vi "Test2_3a.vi"(7 "Report Enable":bool=TRUE, 8 "error in":errorcluster, 9 "Cycles Burst":i32=10000, 11 "Instrument VISA in":T1={"AWG VISA"="81160A", "Oscilloscope  VISA "="labosc4", "Integration Board IP"="172.16.7.43", "connection ID"=refnum, "report out"=refnum, "report file path"=path "D:/CTA/Data_test/test3a"}) -> (0 "error out":errorcluster, 3 "Instrument VISA out":T1={"AWG VISA"="81160A", "Oscilloscope  VISA "="DSO80204B", "Integration Board IP"="172.16.7.43", "connection ID"=refnum, "report out"=refnum, "report file path"=path "D:/CTA/LevelTriggerBoardTest/TestsData/sumtrigger_delay/dataruben"})   [LabVIEW 2009]
uses:
  <vilib>/Utility/NIReport.llb/NI_report.lvclass
  <vilib>/Utility/NIReport.llb/HTML/NI_HTML.lvclass
  <instrlib>/Agilent 8000 Series/Public/Configure/Configure Math (Binary Operation).vi
  <instrlib>/Agilent 81150/Agilent 81150.lvlib
  <instrlib>/Agilent 8000 Series/Agilent 8000 Series.lvlib
panel:
  in  "Voltages comprobation 2":dbl[](array[numeric])=[0.05, 0.1, 0.2, 0.3, 0.35, 0.4, 0.45, 0.5, 0.55, 0.6, 0.7, 0.8, 0.9, 1.0, 1.2, 1.5, 1.8, 2.0]
  in  "Voltages comprobation":dbl[](array[numeric])=[0.05, 0.1, 0.2, 0.3, 0.35, 0.4, 0.45, 0.5, 0.55, 0.6, 0.7, 0.8, 0.9, 1.0, 1.2, 1.5, 1.8, 2.0]
  in  "cliipping":i32[](array[numeric])=[504, 502, 520, 505, 498, 488, 458]
  in  "attenuation":i32[](array[numeric])=[1473, 1472, 1442, 1475, 1463, 1454, 1478]
  in  "Channels":i32[](array[numeric])=[0, 1, 2, 3, 4, 5, 6]
  in  "Quantity of measurements":u32=10
  in  "Save NOW!":bool
  in  "End 2":bool=TRUE
  out "Data output":dbl[][](array[numeric])=[[1.0, 1.0, 2200.0, 200.0, 0.0, 0.26, nan, 1.00955e-08, nan, 2.8861e-09, nan, 0.961, nan], [1.0, 1.0, 2200.0, 200.0, 1.0, 0.261, nan, 1.0146e-08, nan, 2.9059e-09, nan, 0.961, nan]]
  out "Measurement":dbl=0.261
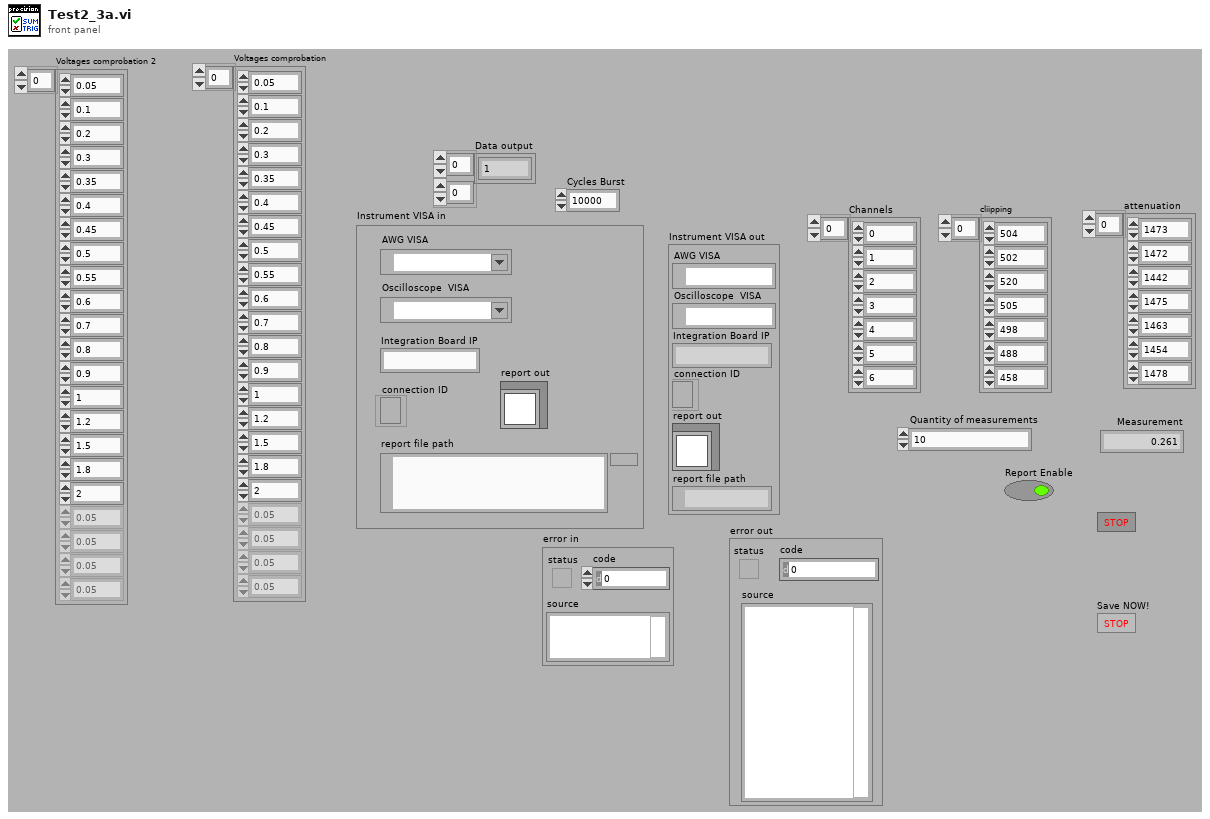
[diagram p1: front panel]
types:
  T1 = cluster{"AWG VISA":refnum<visa-resource-name>, "Oscilloscope  VISA ":refnum<visa-resource-name>, "Integration Board IP":string, "connection ID":refnum<k5>, "report out":refnum<class "NI_report.lvclass">, "report file path":path}
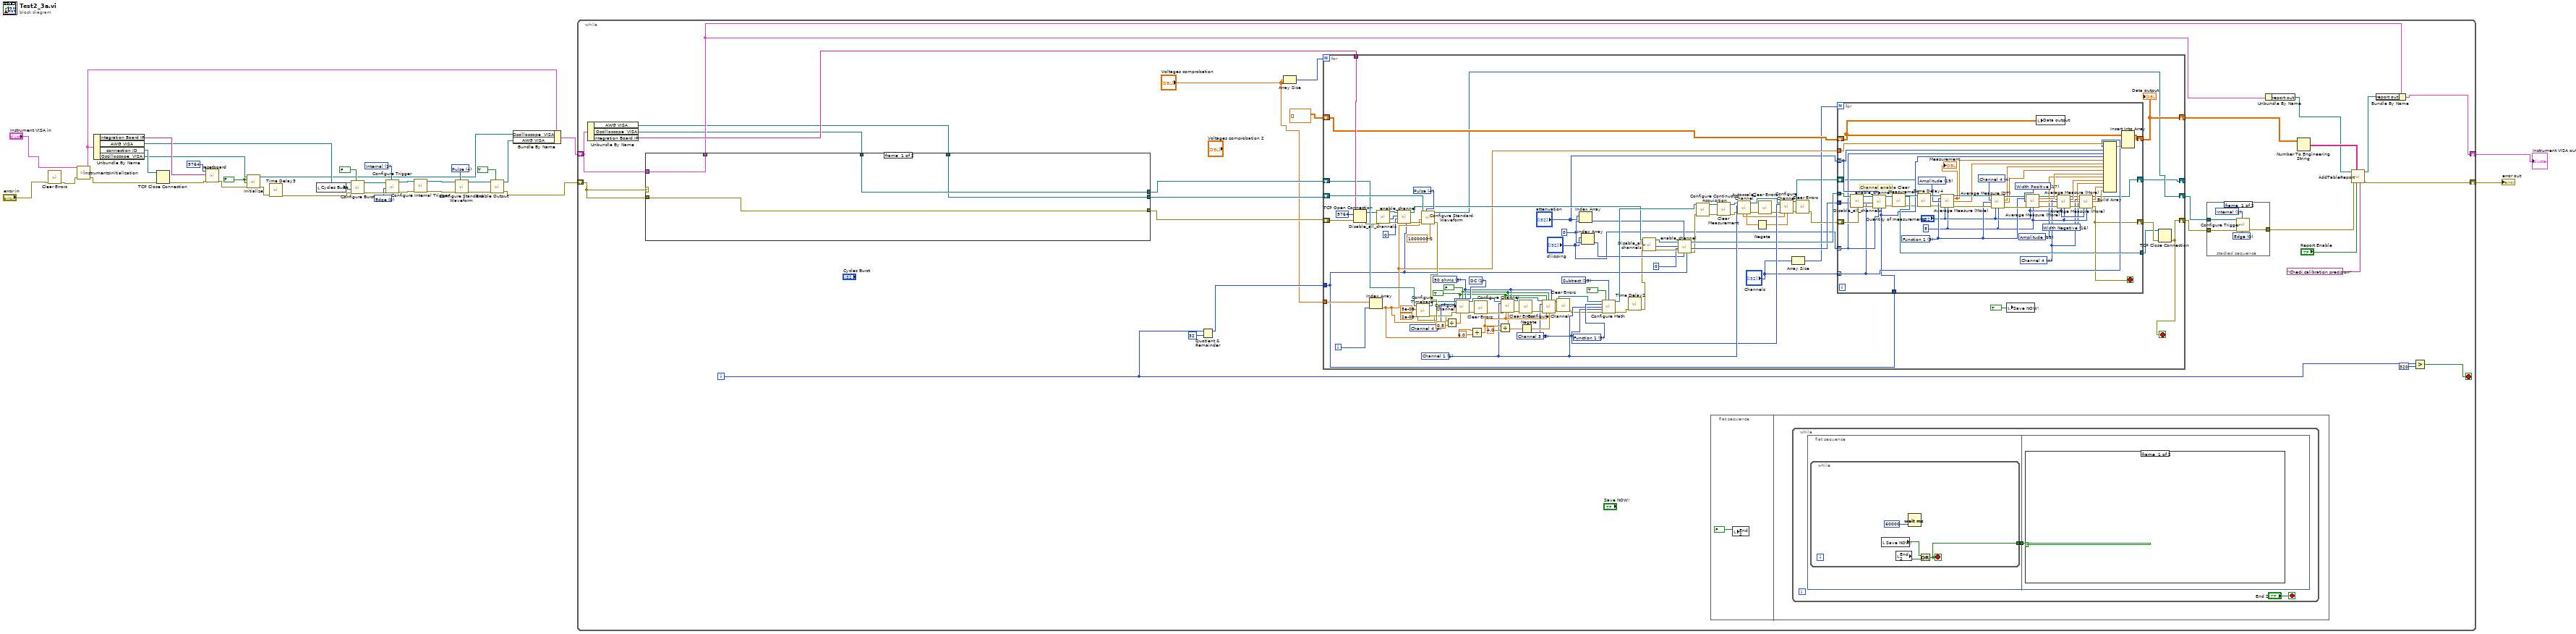
[diagram p0: block diagram]
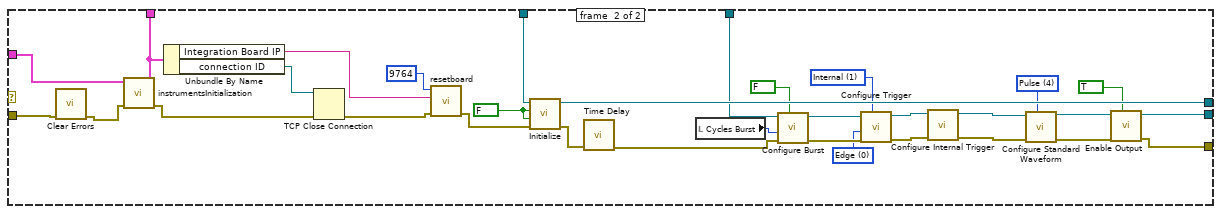
[diagram p2: hidden frame]
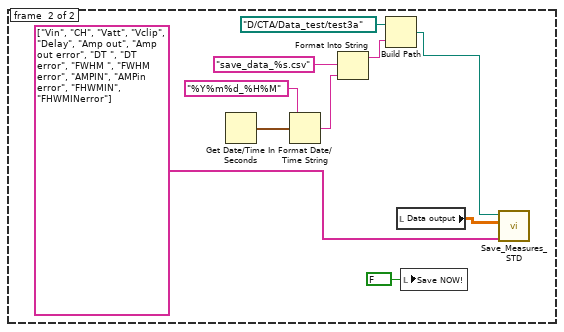
[diagram p3: hidden frame]
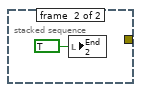
[diagram p4: hidden frame]
diagram:
  w18 = u16 1 items=["Immediate", "Internal", "External", "Software Trigger Function"] ("Trigger Source (0: Immediate)")
  w19 = u16 0 items=["Edge", "Level"] ("Trigger Mode (0: Edge)")
  w26 = u16 4 items=["Sine", "Square", "Ramp Up", "Ramp Down", "Pulse", "Noise", "DC"] ("Waveform (0: Sine)")
  w31 = FALSE ("ID Query (True)")
  n1 = call <vilib>:"Clear Errors.vi"("error in (no error)"="error in") -> ("error out"=w28:errorcluster)  [unwired: 6 in]
  n2 = call "instrumentsInitialization.vi"("error in"=w28, "Instrument VISA in"="Instrument VISA in") -> ("error out"=w11:errorcluster, "Instrument VISA out"=w4:T1)  [unwired: 8 in]
  n3 = Unbundle By Name(w4) -> ("Integration Board IP"=w33:string, "AWG VISA"=w6:refnum<visa-resource-name>, "connection ID"=w12:refnum<k5>, "Oscilloscope  VISA"=w7:refnum<visa-resource-name>)
  n4 = TCP Close Connection(connection ID=w12, error in (no error)=w11) -> (error out=w10:errorcluster)  [unwired: 1 in, 1 out]
  n5 = call "resetboard.vi"("error in (no error)"=w10, "address"=w33, "remote port or service name"=u16 9764) -> ("error out"=w30:errorcluster)  [unwired: 7 in, 1 out]
  n6 = call <instrlib>:"Initialize.vi"("error in (no error)"=w30, "Reset (True)"=w31, "ID Query (True)"=w31, "VISA resource name"=w7) -> ("error out"=w29:errorcluster, "VISA resource name out"=w3:refnum<visa-resource-name>)  [unwired: 6 in]
  n7 = call "Time Delay3"("error in (no error)"=w29) -> ("error out"=w13:errorcluster)  [unwired: 10 in]
  n8 = local read "Cycles Burst"() -> (w22:i32)
  n9 = call <instrlib>:"Configure Burst.vi"("Enable Burst (F: Disable)"=FALSE, "error in (no error)"=w13, "Burst Count (2)"=w22, "VISA resource name"=w6) -> ("error out"=w21:errorcluster, "VISA resource name out"=w20:refnum<visa-resource-name>)  [unwired: 6 in]
  n10 = call <instrlib>:"Configure Trigger.vi"("Trigger Source (0: Immediate)"=w18, "error in (no error)"=w21, "Trigger Mode (0: Edge)"=w19, "VISA resource name"=w20) -> ("error out"=w17:errorcluster, "VISA resource name out"=w16:refnum<visa-resource-name>)  [unwired: 6 in]
  n11 = call <instrlib>:"Configure Internal Trigger.vi"("error in (no error)"=w17, "VISA resource name"=w16) -> ("error out"=w14:errorcluster, "VISA resource name out"=w15:refnum<visa-resource-name>)  [unwired: 8 in]
  n12 = call <instrlib>:"Configure Standard Waveform.vi"("Waveform (0: Sine)"=w26, "error in (no error)"=w14, "VISA resource name"=w15) -> ("error out"=w25:errorcluster, "VISA resource name out"=w24:refnum<visa-resource-name>)  [unwired: 7 in]
  n13 = call <instrlib>:"Enable Output.vi"("Enable Output (T: Enable)"=TRUE, "error in (no error)"=w25, "VISA resource name"=w24) -> ("error out"=w5:errorcluster, "VISA resource name out"=w2:refnum<visa-resource-name>)  [unwired: 7 in]
  n14 = Bundle By Name(cluster=w4, "Oscilloscope  VISA"=w3, "AWG VISA"=w2) -> (w1:T1)
  n15 = while {
    shift-right: [w48] -> w35
    shift-left: w5 -> [w40]
    shift-right: [w44] -> w34
    shift-left: w1 -> [w46]
    i -> [w51]
    stop <- w53 stop-if-true
    n16 = Unbundle By Name(w46) -> ("AWG VISA"=w39:refnum<visa-resource-name>, "Oscilloscope  VISA"=w42:refnum<visa-resource-name>, "Integration Board IP"=w47:string)
    n17 = case shown="Error" w40 {
      tunnel: w46 -> [w67 w99]
      tunnel: w40 -> [w66 w90]
      tunnel: [w67 w98] -> w45
      tunnel: [w66 w72] -> w37
      tunnel: w42 -> [w65 w95]
      tunnel: [w65 w94] -> w41
      tunnel: w39 -> [w64 w74]
      tunnel: [w64 w73] -> w38
      frame #0 {
      }
      frame #1 {
        w79 = u16 1 items=["Immediate", "Internal", "External", "Software Trigger Function"] ("Trigger Source (0: Immediate)")
        w80 = u16 0 items=["Edge", "Level"] ("Trigger Mode (0: Edge)")
        w87 = u16 4 items=["Sine", "Square", "Ramp Up", "Ramp Down", "Pulse", "Noise", "DC"] ("Waveform (0: Sine)")
        w93 = FALSE ("ID Query (True)")
        n18 = call <vilib>:"Clear Errors.vi"("error in (no error)"=w90) -> ("error out"=w89:errorcluster)  [unwired: 6 in]
        n19 = call "instrumentsInitialization.vi"("error in"=w89, "Instrument VISA in"=w99) -> ("error out"=w69:errorcluster, "Instrument VISA out"=w98:T1)  [unwired: 8 in]
        n20 = Unbundle By Name(w98) -> ("Integration Board IP"=w97:string, "connection ID"=w70:refnum<k5>)
        n21 = TCP Close Connection(connection ID=w70, error in (no error)=w69) -> (error out=w68:errorcluster)  [unwired: 1 in, 1 out]
        n22 = call "resetboard.vi"("error in (no error)"=w68, "address"=w97, "remote port or service name"=u16 9764) -> ("error out"=w92:errorcluster)  [unwired: 7 in, 1 out]
        n23 = call <instrlib>:"Initialize.vi"("error in (no error)"=w92, "Reset (True)"=w93, "ID Query (True)"=w93, "VISA resource name"=w95) -> ("error out"=w91:errorcluster, "VISA resource name out"=w94:refnum<visa-resource-name>)  [unwired: 6 in]
        n24 = call "Time Delay"("error in (no error)"=w91) -> ("error out"=w71:errorcluster)  [unwired: 10 in]
        n25 = local read "Cycles Burst"() -> (w83:i32)
        n26 = call <instrlib>:"Configure Burst.vi"("Enable Burst (F: Disable)"=FALSE, "error in (no error)"=w71, "Burst Count (2)"=w83, "VISA resource name"=w74) -> ("error out"=w82:errorcluster, "VISA resource name out"=w81:refnum<visa-resource-name>)  [unwired: 6 in]
        n27 = call <instrlib>:"Configure Trigger.vi"("Trigger Source (0: Immediate)"=w79, "error in (no error)"=w82, "Trigger Mode (0: Edge)"=w80, "VISA resource name"=w81) -> ("error out"=w78:errorcluster, "VISA resource name out"=w77:refnum<visa-resource-name>)  [unwired: 6 in]
        n28 = call <instrlib>:"Configure Internal Trigger.vi"("error in (no error)"=w78, "VISA resource name"=w77) -> ("error out"=w75:errorcluster, "VISA resource name out"=w76:refnum<visa-resource-name>)  [unwired: 8 in]
        n29 = call <instrlib>:"Configure Standard Waveform.vi"("Waveform (0: Sine)"=w87, "error in (no error)"=w75, "VISA resource name"=w76) -> ("error out"=w86:errorcluster, "VISA resource name out"=w85:refnum<visa-resource-name>)  [unwired: 7 in]
        n30 = call <instrlib>:"Enable Output.vi"("Enable Output (T: Enable)"=TRUE, "error in (no error)"=w86, "VISA resource name"=w85) -> ("error out"=w72:errorcluster, "VISA resource name out"=w73:refnum<visa-resource-name>)  [unwired: 7 in]
      }
    }
    n31 = Quotient & Remainder(x=w51, y=32) -> (x-y*floor(x/y)=w49:i32)  [unwired: 1 out]
    n32 = Array Size(array="Voltages comprobation") -> (size(s)=w54:i32)
    n33 = for {
      N: w54 -> [_]
      shift-right: [w204] -> w63
      shift-left: w37 -> [w207]
      tunnel: w47 -> [w206]
      shift-right: [w164] -> w58
      shift-left: dbl[][] [] -> [w167]
      tunnel: "Voltages comprobation" -> [w163]
      tunnel: w49 -> [w132]
      shift-right: [w131] -> w43
      shift-left: w38 -> [w210]
      shift-right: [w130] -> _
      shift-left: w41 -> [w201]
      i -> [w209]
      stop <- w204 stop-if-true
      w139 = 0 ("index")
      w181 = TRUE ("Enable Channel (Enable)")
      w183 = FALSE ("BW Limit 20MHz (Disable)")
      w182 = u32 0 items=["50 ohms", "1 Mohms"] ("Input Impedance (1: 1 Mohms)")
      w191 = 4 items=["Channel 1"=1, "Channel 2"=2, "Channel 3"=3, "Channel 4"=4] ("Channel (1: Channel 1)")
      w192 = 1 items=["AC", "DC"] ("Vertical Coupling (1: DC)")
      w196 = u16 5 items=["Function 1"=5, "Function 2"=6, "Function 3"=7, "Function 4"=8] ("Math Channel (5: Function 1)")
      w197 = u16 15 items=["Add"=12, "Divide"=13, "Multiply"=14, "Subtract"=15, "Common Mode"=16, "Versus"=17] ("Math Operation (12: Add)")
      w166 = 1 items=["Channel 1"=1, "Channel 2"=2, "Channel 3"=3, "Channel 4"=4] ("Channel (1: Channel 1)")
      w165 = 3 items=["Channel 1"=1, "Channel 2"=2, "Channel 3"=3, "Channel 4"=4] ("Channel (1: Channel 1)")
      w211 = u16 4 items=["Sine", "Square", "Ramp Up", "Ramp Down", "Pulse", "Noise", "DC"] ("Waveform (0: Sine)")
      n34 = TCP Open Connection(address=w206, remote port or service name=u16 9764, error in (no error)=w207) -> (connection ID=w178:refnum<k5>, error out=w179:errorcluster)  [unwired: 2 in]
      n35 = Index Array(array=w163, index=w209) -> (element=w162:dbl)
      n36 = call "Disable_all_channels.vi"("error in"=w179, "connection ID"=w178) -> ("error out"=w174:errorcluster, "id_out"=w173:i32, "connection ID out"=w176:refnum<k5>)  [unwired: 7 in]
      n37 = call "enable_channel.vi"("Delay"=w132, "error in"=w174, "Channel"=u16 0 ("remote port or service name"), "id_in"=w173, "connection ID"=w176) -> ("error out"=w175:errorcluster, "connection ID out"=w177:refnum<k5>)  [unwired: 4 in, 1 out]
      n38 = call <instrlib>:"Configure Standard Waveform.vi"("Frequency (1000.0 Hz)"=1000000.0, "Waveform (0: Sine)"=w211, "error in (no error)"=w175, "Amplitude (1.0 Vpp)"=w162, "VISA resource name"=w210) -> ("error out"=w200:errorcluster, "VISA resource name out"=w131:refnum<visa-resource-name>)  [unwired: 5 in]
      n39 = call <instrlib>:"Configure Timebase.vi"("error in (no error)"=w200, "Position (0.0 s)"=2e-08, "Timebase (0.005 s)"=5e-08, "VISA resource name"=w201) -> ("error out"=w193:errorcluster, "VISA resource name out"=w194:refnum<visa-resource-name>)  [unwired: 6 in]
      n40 = Divide(x=w162, y=0.5) -> (x/y=w160:dbl)
      n41 = call <instrlib>:"Configure Channel.vi"("VISA resource name"=w194, "Enable Channel (Enable)"=w181, "BW Limit 20MHz (Disable)"=w183, "Input Impedance (1: 1 Mohms)"=w182, "Channel (1: Channel 1)"=w191, "Vertical Coupling (1: DC)"=w192, "error in (no error)"=w193, "Vertical Range (2.0 V)"=w160) -> ("VISA resource name out"=w189:refnum<visa-resource-name>, "error out"=w190:errorcluster)  [unwired: 6 in]
      n42 = Divide(x=w162, y=6.0) -> (x/y=w171:dbl)
      n43 = call <vilib>:"Clear Errors.vi"("error in (no error)"=w190) -> ("error out"=w186:errorcluster)  [unwired: 6 in]
      n44 = Divide(x=w171, y=4.0) -> (x/y=w168:dbl)
      n45 = call <instrlib>:"Configure Channel.vi"("VISA resource name"=w189, "Enable Channel (Enable)"=w181, "BW Limit 20MHz (Disable)"=w183, "Input Impedance (1: 1 Mohms)"=w182, "Channel (1: Channel 1)"=w166, "error in (no error)"=w186, "Vertical Range (2.0 V)"=w171, "Vertical Offset (0.0 V)"=w168) -> ("VISA resource name out"=w188:refnum<visa-resource-name>, "error out"=w185:errorcluster)  [unwired: 6 in]
      n46 = call <vilib>:"Clear Errors.vi"("error in (no error)"=w185) -> ("error out"=w184:errorcluster)  [unwired: 6 in]
      n47 = Negate(x=w168) -> (-x=w169:dbl)
      n48 = call <instrlib>:"Configure Channel.vi"("VISA resource name"=w188, "Enable Channel (Enable)"=w181, "BW Limit 20MHz (Disable)"=w183, "Input Impedance (1: 1 Mohms)"=w182, "Channel (1: Channel 1)"=w165, "error in (no error)"=w184, "Vertical Range (2.0 V)"=w171, "Vertical Offset (0.0 V)"=w169) -> ("VISA resource name out"=w187:refnum<visa-resource-name>, "error out"=w126:errorcluster)  [unwired: 6 in]
      n49 = call <vilib>:"Clear Errors.vi"("error in (no error)"=w126) -> ("error out"=w125:errorcluster)  [unwired: 6 in]
      n50 = Index Array(array="attenuation", index=w139) -> (element=w137:i32)
      n51 = Index Array(array="cliipping", index=w139) -> (element=w138:i32)
      n52 = call-poly <instrlib>:"Configure Math.vi"("VISA resource name"=w187, "Enable Math Channel (T:Enable)"=TRUE, "Math Operation (12: Add)"=w197, "Math Channel (5: Function 1)"=w196, "Math Operand (1: Channel 1)"=w166, "Math Operand (2: Channel 2)"=w165, "error in (no error)"=w125) -> ("VISA resource name out"=w199:refnum<visa-resource-name>, "error out"=w127:errorcluster)  [unwired: 7 in]
      n53 = call "Time Delay2"("error in (no error)"=w127) -> ("error out"=w128:errorcluster)  [unwired: 10 in]
      n54 = call "Disable_all_channels.vi"("error in"=w128, "connection ID"=w177) -> ("error out"=w159:errorcluster, "id_out"=w156:i32, "connection ID out"=w158:refnum<k5>)  [unwired: 7 in]
      n55 = call "enable_channel.vi"("Delay"=w132, "V clip"=w138, "V att"=w137, "error in"=w159, "Channel"=u32 0 ("Max Errors"), "id_in"=w156, "connection ID"=w158) -> ("error out"=w143:errorcluster, "id_out"=w154:i32, "connection ID out"=w157:refnum<k5>)  [unwired: 2 in]
      n56 = call <instrlib>:"Configure Continuous Acquisition.vi"("error in (no error)"=w143, "VISA resource name"=w199) -> ("error out"=w142:errorcluster, "VISA resource name out"=w144:refnum<visa-resource-name>)  [unwired: 8 in]
      n57 = call <instrlib>:"Clear Measurement.vi"("error in (no error)"=w142, "VISA resource name"=w144) -> ("error out"=w146:errorcluster, "VISA resource name out"=w145:refnum<visa-resource-name>)  [unwired: 8 in]
      n58 = call "Autoscale_Channel.vi"("error in"=w146, "Channel"=w166, "VISA resource name"=w145) -> ("error out"=w148:errorcluster, "VISA resource name out"=w153:refnum<visa-resource-name>, "Offset"=w133:dbl, "VerticalRange"=w152:dbl)  [unwired: 5 in]
      n59 = Negate(x=w133) -> (-x=w134:dbl)
      n60 = call <vilib>:"Clear Errors.vi"("error in (no error)"=w148) -> ("error out"=w149:errorcluster)  [unwired: 6 in]
      n61 = call <instrlib>:"Configure Channel.vi"("VISA resource name"=w153, "Channel (1: Channel 1)"=w165, "error in (no error)"=w149, "Vertical Range (2.0 V)"=w152, "Vertical Offset (0.0 V)"=w134) -> ("VISA resource name out"=w129:refnum<visa-resource-name>, "error out"=w150:errorcluster)  [unwired: 9 in]
      n62 = Array Size(array="Channels") -> (size(s)=w140:i32)
      n63 = call <vilib>:"Clear Errors.vi"("error in (no error)"=w150) -> ("error out"=w151:errorcluster)  [unwired: 6 in]
      n64 = for {
        N: w140 -> [_]
        shift-right: [w225] -> w205
        shift-left: w151 -> [w258]
        tunnel: w157 -> [w259]
        tunnel: [w261] -> w203
        tunnel: w162 -> [w255]
        shift-right: [w253] -> w164
        shift-left: w167 -> [w235]
        tunnel: "attenuation" -> [w238] mode=indexing
        tunnel: "cliipping" -> [w237] mode=indexing
        tunnel: w154 -> [w236]
        tunnel: "Channels" -> [w229] mode=indexing
        tunnel: w132 -> [w227]
        shift-right: [w217] -> w130
        shift-left: w129 -> [w216]
        stop <- w225 stop-if-true
        w218 = 16 items=["Rise Time", "Fall Time", "Frequency", "Period", "Voltage RMS(AC)", "Voltage RMS(DC)", "Voltage RMS (AC,cycle)", "Voltage RMS (DC,cycle)", "Voltage Max", "Voltage Min", "Voltage Middle", "Voltage Vpp", "Voltage High", "Voltage Low", "Voltage Average", "Voltage Average (cycle)", "Width Negative", "Width Positive", "Duty Cycle Positive", "Amplitude", "Overshoot", "Preshoot", "Voltage Base", "Voltage Upper", "Time Max", "Time Min", "Color Grade Crossing", "Color Grade Eye Width", "Color Grade Eye Height", "Color Grade Eye Q-Factory", "Color Grade Eye Duty Cycle Distortion(Percent)", "Color Grade Eye Duty Cycle Distortion(Time)", "Color Grade Eye Jitter(PP)", "Color Grade Eye Width(RMS)", "Cycle-cycle Duty Jitter(Rising)", "Cycle-cycle Duty Jitter(Falling)", "Cycle-cycle Jitter(Rising)", "Cycle-cycle Jitter(Falling)", "Cycle-cycle - Width", "Cycle-cycle + Width", "Date Rate", "Unit Interval", "FFT Delta Frequency", "FFT Delta Magnitude", "FFT Frequency", "FFT Magnitude", "Slew Rate", "Area (Entire Display)", "Area(Single Cycle)", "Duty Cycle (Rising)", "Duty Cycle (Falling)"] ("Measurement Function (0: Rise Time)")
        w219 = 4 items=["Channel 1"=1, "Channel 2"=2, "Channel 3"=3, "Channel 4"=4, "Function 1"=5, "Function 2"=6, "Function 3"=7, "Function 4"=8, "Memory 1"=9, "Memory 2"=10, "Memory 3"=11, "Memory 4"=12] ("Channel (1: Channel 1)")
        w233 = 19 items=["Rise Time", "Fall Time", "Frequency", "Period", "Voltage RMS(AC)", "Voltage RMS(DC)", "Voltage RMS (AC,cycle)", "Voltage RMS (DC,cycle)", "Voltage Max", "Voltage Min", "Voltage Middle", "Voltage Vpp", "Voltage High", "Voltage Low", "Voltage Average", "Voltage Average (cycle)", "Width Negative", "Width Positive", "Duty Cycle Positive", "Amplitude", "Overshoot", "Preshoot", "Voltage Base", "Voltage Upper", "Time Max", "Time Min", "Color Grade Crossing", "Color Grade Eye Width", "Color Grade Eye Height", "Color Grade Eye Q-Factory", "Color Grade Eye Duty Cycle Distortion(Percent)", "Color Grade Eye Duty Cycle Distortion(Time)", "Color Grade Eye Jitter(PP)", "Color Grade Eye Width(RMS)", "Cycle-cycle Duty Jitter(Rising)", "Cycle-cycle Duty Jitter(Falling)", "Cycle-cycle Jitter(Rising)", "Cycle-cycle Jitter(Falling)", "Cycle-cycle - Width", "Cycle-cycle + Width", "Date Rate", "Unit Interval", "FFT Delta Frequency", "FFT Delta Magnitude", "FFT Frequency", "FFT Magnitude", "Slew Rate", "Area (Entire Display)", "Area(Single Cycle)", "Duty Cycle (Rising)", "Duty Cycle (Falling)"] ("Measurement Function (0: Rise Time)")
        w221 = u32 5 ("Max Errors")
        w249 = 17 items=["Rise Time", "Fall Time", "Frequency", "Period", "Voltage RMS(AC)", "Voltage RMS(DC)", "Voltage RMS (AC,cycle)", "Voltage RMS (DC,cycle)", "Voltage Max", "Voltage Min", "Voltage Middle", "Voltage Vpp", "Voltage High", "Voltage Low", "Voltage Average", "Voltage Average (cycle)", "Width Negative", "Width Positive", "Duty Cycle Positive", "Amplitude", "Overshoot", "Preshoot", "Voltage Base", "Voltage Upper", "Time Max", "Time Min", "Color Grade Crossing", "Color Grade Eye Width", "Color Grade Eye Height", "Color Grade Eye Q-Factory", "Color Grade Eye Duty Cycle Distortion(Percent)", "Color Grade Eye Duty Cycle Distortion(Time)", "Color Grade Eye Jitter(PP)", "Color Grade Eye Width(RMS)", "Cycle-cycle Duty Jitter(Rising)", "Cycle-cycle Duty Jitter(Falling)", "Cycle-cycle Jitter(Rising)", "Cycle-cycle Jitter(Falling)", "Cycle-cycle - Width", "Cycle-cycle + Width", "Date Rate", "Unit Interval", "FFT Delta Frequency", "FFT Delta Magnitude", "FFT Frequency", "FFT Magnitude", "Slew Rate", "Area (Entire Display)", "Area(Single Cycle)", "Duty Cycle (Rising)", "Duty Cycle (Falling)"] ("Measurement Function (0: Rise Time)")
        w240 = u16 4 items=["Channel 1"=1, "Channel 2"=2, "Channel 3"=3, "Channel 4"=4, "Function 1"=5, "Function 2"=6, "Function 3"=7, "Function 4"=8, "Memory 1"=9, "Memory 2"=10, "Memory 3"=11, "Memory 4"=12] ("Channel1 (1: Channel 1)")
        w239 = 5 items=["Channel 1"=1, "Channel 2"=2, "Channel 3"=3, "Channel 4"=4, "Function 1"=5, "Function 2"=6, "Function 3"=7, "Function 4"=8, "Memory 1"=9, "Memory 2"=10, "Memory 3"=11, "Memory 4"=12] ("aa")
        w250 = 19 items=["Rise Time", "Fall Time", "Frequency", "Period", "Voltage RMS(AC)", "Voltage RMS(DC)", "Voltage RMS (AC,cycle)", "Voltage RMS (DC,cycle)", "Voltage Max", "Voltage Min", "Voltage Middle", "Voltage Vpp", "Voltage High", "Voltage Low", "Voltage Average", "Voltage Average (cycle)", "Width Negative", "Width Positive", "Duty Cycle Positive", "Amplitude", "Overshoot", "Preshoot", "Voltage Base", "Voltage Upper", "Time Max", "Time Min", "Color Grade Crossing", "Color Grade Eye Width", "Color Grade Eye Height", "Color Grade Eye Q-Factory", "Color Grade Eye Duty Cycle Distortion(Percent)", "Color Grade Eye Duty Cycle Distortion(Time)", "Color Grade Eye Jitter(PP)", "Color Grade Eye Width(RMS)", "Cycle-cycle Duty Jitter(Rising)", "Cycle-cycle Duty Jitter(Falling)", "Cycle-cycle Jitter(Rising)", "Cycle-cycle Jitter(Falling)", "Cycle-cycle - Width", "Cycle-cycle + Width", "Date Rate", "Unit Interval", "FFT Delta Frequency", "FFT Delta Magnitude", "FFT Frequency", "FFT Magnitude", "Slew Rate", "Area (Entire Display)", "Area(Single Cycle)", "Duty Cycle (Rising)", "Duty Cycle (Falling)"] ("Measurement Function (0: Rise Time)")
        # "Channel enable"
        n65 = call "Disable_all_channels.vi"("error in"=w258, "id_in"=w236, "connection ID"=w259) -> ("error out"=w257:errorcluster, "id_out"=w256:i32, "connection ID out"=w260:refnum<k5>)  [unwired: 6 in]
        n66 = call "enable_channel.vi"("Delay"=w227, "V clip"=w237, "V att"=w238, "error in"=w257, "Channel"=w229, "id_in"=w256, "connection ID"=w260) -> ("error out"=w215:errorcluster, "connection ID out"=w261:refnum<k5>)  [unwired: 2 in, 1 out]
        n67 = call <instrlib>:"Clear Measurement.vi"("error in (no error)"=w215, "VISA resource name"=w216) -> ("error out"=w213:errorcluster, "VISA resource name out"=w251:refnum<visa-resource-name>)  [unwired: 8 in]
        n68 = call "Time Delay4"("error in (no error)"=w213) -> ("error out"=w214:errorcluster)  [unwired: 10 in]
        n69 = call "Average Measure (More).vi"("VISA resource name"=w251, "Channel (1: Channel 1)"=w239, "Measurement Function (0: Rise Time)"=w250, "error in (no error)"=w214, "Averages"="Quantity of measurements", "Max Errors"=w221) -> ("VISA resource name out"=w248:refnum<visa-resource-name>, "Measure Average"=w228:dbl, "Measure Error"=w252:dbl, "error out"=w245:errorcluster)  [unwired: 6 in]
        "Measurement" <- w228
        n70 = call "Average Measure (DT).vi"("VISA resource name"=w248, "Channel1 (1: Channel 1)"=w240, "Channel2 (2: Channel 2)"=w239, "error in (no error)"=w245, "Averages"="Quantity of measurements", "Max Errors"=w221) -> ("VISA resource name out"=w247:refnum<visa-resource-name>, "Measure Average"=w244:dbl, "Measure Error"=w243:dbl, "error out"=w246:errorcluster)  [unwired: 6 in]
        n71 = call "Average Measure (More).vi"("VISA resource name"=w247, "Channel (1: Channel 1)"=w239, "Measurement Function (0: Rise Time)"=w249, "error in (no error)"=w246, "Averages"="Quantity of measurements", "Max Errors"=w221) -> ("VISA resource name out"=w232:refnum<visa-resource-name>, "Measure Average"=w242:dbl, "Measure Error"=w241:dbl, "error out"=w234:errorcluster)  [unwired: 6 in]
        n72 = local write "Data output"(w235) -> ()
        n73 = call "Average Measure (More).vi"("VISA resource name"=w232, "Channel (1: Channel 1)"=w219, "Measurement Function (0: Rise Time)"=w233, "error in (no error)"=w234, "Averages"="Quantity of measurements", "Max Errors"=w221) -> ("VISA resource name out"=w220:refnum<visa-resource-name>, "Measure Average"=w231:dbl, "Measure Error"=w230:dbl, "error out"=w226:errorcluster)  [unwired: 6 in]
        n74 = call "Average Measure (More).vi"("VISA resource name"=w220, "Channel (1: Channel 1)"=w219, "Measurement Function (0: Rise Time)"=w218, "error in (no error)"=w226, "Averages"="Quantity of measurements", "Max Errors"=w221) -> ("VISA resource name out"=w217:refnum<visa-resource-name>, "Measure Average"=w224:dbl, "Measure Error"=w223:dbl, "error out"=w225:errorcluster)  [unwired: 6 in]
        n75 = Build Array(w255, w229, w238, w237, w227, w228, w252, w244, w243, w242, w241, w231, w230, w224, w223) -> (w254:dbl[])
        n76 = Insert Into Array(array=w235, new element=w254) -> (w253:dbl[][])  [unwired: 2 in]
      }
      "Data output" <- w164
      n77 = local write "Save NOW!"(TRUE ("Save NOW! 2")) -> ()
      n78 = TCP Close Connection(connection ID=w203, error in (no error)=w205) -> (error out=w204:errorcluster)  [unwired: 1 in, 1 out]
    }
    n79 = flat-sequence {
      frame #0 {
        n80 = local write "End 2"(FALSE ("End")) -> ()
      }
      frame #1 {
        n81 = while {
          stop <- "End 2" stop-if-true
          n82 = flat-sequence {
            tunnel: [w103] -> w101
            tunnel: w101 -> [w108]
            frame #0 {
              n83 = while {
                tunnel: [w104] -> w103
                stop <- w104 stop-if-true
                n84 = local read "Save NOW!"() -> (w105:bool)
                n85 = local read "End 2"() -> (w106:bool)
                n86 = Wait (ms)(milliseconds to wait=u32 60000) -> ()  [unwired: 1 out]
                n87 = Or(x=w105, y=w106) -> (x .or. y?=w104:bool)
              }
            }
            frame #1 {
              n88 = case shown="True" w108 {
                frame #0 {
                }
                frame #1 {
                  n89 = Get Date/Time In Seconds() -> (seconds since 1Jan1904=w117:timestamp)
                  n90 = Format Date/Time String(time format string (%c)="%Y%m%d_%H%M", seconds (now)=w117) -> (date/time string=w115:string)  [unwired: 1 in]
                  n91 = Format Into String(format string="save_data_%s.csv", w115) -> (resulting string=w114:string)  [unwired: 2 in, 1 out]
                  n92 = Build Path(base path=path "D:/CTA/Data_test/test3a", name or relative path=w114) -> (appended path=w113:path)
                  n93 = local read "Data output"() -> (w110:dbl[][])
                  n94 = local write "Save NOW!"(FALSE ("Save NOW!")) -> ()
                  n95 = call "Save_Measures_STD.vi"("appended array"=string[] ["Vin", "CH", "Vatt", "Vclip", "Delay", "Amp out", "Amp out error", "DT ", "DT error", "FWHM ", "FWHM error", "AMPIN", "AMPin error", "FHWMIN", "FHWMINerror"], "Data in"=w110, "file path (dialog if empty)"=w113) -> ()  [unwired: 9 in]
                }
              }
            }
          }
        }
      }
    }
    n96 = stacked-sequence {
      tunnel: w63 -> [w121 _]
      tunnel: [w120 _] -> w59
      tunnel: w43 -> [w119 _]
      frame #0 {
        w122 = u16 1 items=["Immediate", "Internal", "External", "Software Trigger Function"] ("Trigger Source (0: Immediate)")
        w123 = u16 0 items=["Edge", "Level"] ("Trigger Mode (0: Edge)")
        n97 = call <instrlib>:"Configure Trigger.vi"("Trigger Source (0: Immediate)"=w122, "error in (no error)"=w121, "Trigger Mode (0: Edge)"=w123, "VISA resource name"=w119) -> ("error out"=w120:errorcluster)  [unwired: 6 in, 1 out]
      }
      frame #1 {
        n98 = local write "End 2"(TRUE ("End 2")) -> ()
      }
    }
    n99 = Unbundle By Name(w45) -> ("report out"=w55:refnum<class "NI_report.lvclass">)
    n100 = Number To Engineering String(4:w58) -> (0:w56:string[][])  [unwired: 3 in]
    n101 = call "AddTableReport.vi"("Table title"="Check calibration precision", "Report Enable"="Report Enable", "Data"=w56, "error in"=w59, "report in"=w55) -> ("error out"=w48:errorcluster, "report out"=w60:refnum<class "NI_report.lvclass">)  [unwired: 5 in]
    n102 = Bundle By Name(cluster=w45, "report out"=w60) -> (w44:T1)
    n103 = Greater?(x=w51, y=320) -> (0:w53:bool)
  }
  "Instrument VISA out" <- w34
  "error out" <- w35
